vi "CloseChannelsAll.vi"(2 "error in (no error)":errorcluster) -> (0 "error out":errorcluster)   [LabVIEW 2009]
doc: "Execute a SCPI close for all channels associated with the 6-port switches S1, S2, S3, S4, s5"
panel:
  in  "SCPI commands":string="rout:clos (@5101:5166)\nrout:clos (@7101:7106)\n"
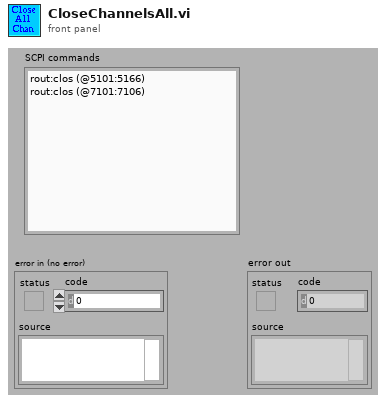
[diagram p1: front panel]
types:
  T1 = enum16{"N1911A", "Siggen", "34980a", "E4418B", "Rvp8"}
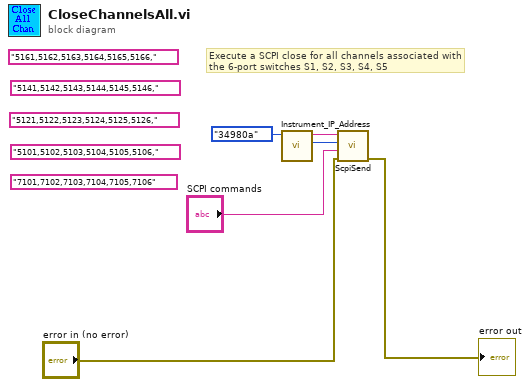
[diagram p0: block diagram]
diagram:
  (unwired) "7101,7102,7103,7104,7105,7106"
  (unwired) "5101,5102,5103,5104,5105,5106,"
  (unwired) "5121,5122,5123,5124,5125,5126,"
  (unwired) "5141,5142,5143,5144,5145,5146,"
  (unwired) "5161,5162,5163,5164,5165,5166,"
  # "Execute a SCPI close for all channels associated with the 6-port switches S1, S2, S3, S4, S5"
  n1 = call "Instrument_IP_Address.vi"("Instrument"=T1."34980a") -> ("Port"=w2:u16, "IP Address"=w3:string)  [unwired: 9 in]
  n2 = call "ScpiSend.vi"("error in (no error)"="error in (no error)", "Command"="SCPI commands", "TCP port"=w2, "IP Address"=w3) -> ("error out"=→"error out":errorcluster)  [unwired: 7 in]
